vi "testGetNotifierServerStatus_tel.vi"(8 "error in (no error)":errorcluster) -> (0 "error out":errorcluster)   [LabVIEW 2018]
uses:
  src/TcpServer/TcpServer.lvclass
  src/TcpServer/TcpServer.lvclass/TcpServer.ctl
  src/TcpServerBase/TcpServerBase.lvclass/TcpServerBase.ctl
  src/TcpServerTel/TcpServerTel.lvclass
  home/pcortes/Documents/github/ts_labview_tcp_json/src/TcpServerBase/TcpServerBase.lvclass
  <vilib>/addons/_JKI Toolkits/Caraya/classes/Assert/Assert Equal Type_Variant.vi
  <vilib>/addons/_JKI Toolkits/Caraya/classes/Test/Test.lvclass
  <vilib>/addons/_JKI Toolkits/Caraya/classes/Assert/Assert.lvclass
  src/TcpServerBase/TcpServerBase.lvclass
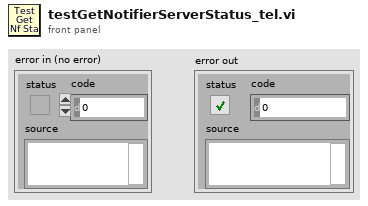
[diagram p1: front panel]
types:
  T1 = cluster{"connectionStatus":bool, "errorSource":string}
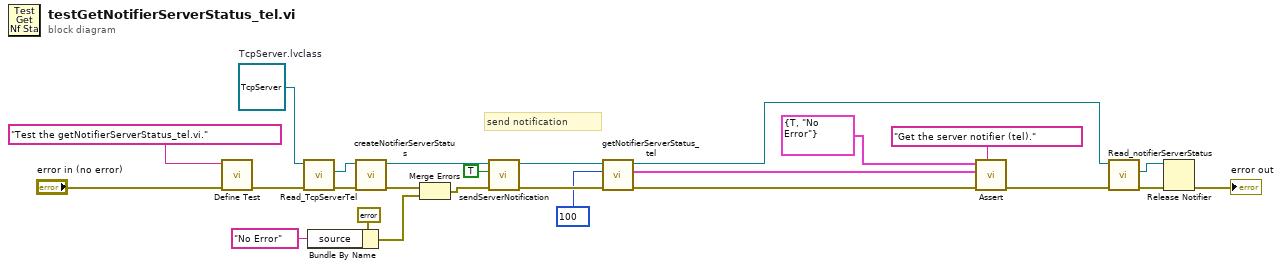
[diagram p0: block diagram]
diagram:
  w13 = refnum<class "TcpServer.lvclass"> refnum  # TcpServer.lvclass
  # "send notification"
  n1 = call <vilib>:"Define Test.vi"("error in (no error)"="error in (no error)", "Label (VI Title)"="Test the getNotifierServerStatus_tel.vi.") -> ("error out"=w10:errorcluster)  [unwired: 9 in]
  n2 = call "Read_TcpServerTel.vi"("error in (no error)"=w10, "TcpServer in"=w13) -> ("error out"=w11:errorcluster, "TcpServerTel.lvclass"=w12:refnum<class "TcpServerTel.lvclass">)  [unwired: 7 in, 1 out]
  n3 = Bundle By Name(cluster=errorcluster {"status"=FALSE, "code"=0, "source"=""} ("error in (no error)"), "source"="No Error") -> (w16:errorcluster)
  n4 = call "createNotifierServerStatus.vi"("error in (no error)"=w11, "tcpServerBase in"=w12) -> ("error out"=w15:errorcluster, "tcpServerBase out"=w22:refnum<class "TcpServerTel.lvclass">)  [unwired: 8 in]
  n5 = Merge Errors(w15, w16) -> (w17:errorcluster)
  n6 = call "sendServerNotification.vi"("error in (no error)"=w17, "connectionStatus"=TRUE ("serverStatus"), "TcpServerBase in"=w22) -> ("error out"=w7:errorcluster, "TcpServerBase out"=w5:refnum<class "TcpServerTel.lvclass">)  [unwired: 7 in]
  n7 = call "getNotifierServerStatus_tel.vi"("error in (no error)"=w7, "Timeout Notifier"=100, "TcpServerTel in"=w5) -> ("error out"=w8:errorcluster, "connStatusCluster"=w9:T1, "TcpServerTel out"=w2:refnum<class "TcpServerTel.lvclass">)  [unwired: 5 in, 1 out]
  n8 = call-poly <vilib>:"Assert.vi"("Label"="Get the server notifier (tel).", "error in (no error)"=w8, "Y"=w9, "X"=T1 {"connectionStatus"=TRUE, "errorSource"="No Error"} ("notification")) -> ("error out"=w14:errorcluster)  [unwired: 7 in]
  n9 = call "Read_notifierServerStatus.vi"("error in (no error)"=w14, "TcpServerBase in"=w2) -> ("error out"=w4:errorcluster, "notifierServerStatus"=w1:refnum<notifier>)  [unwired: 7 in, 1 out]
  n10 = Release Notifier(notifier=w1, error in (no error)=w4) -> (error out=→"error out":errorcluster)  [unwired: 1 in, 2 out]
